vi "Gainsel.vi"(0 "Gain":enum16{"LOW", "HI", "MAX"}(ring)) -> (1 "LO":bool=TRUE, 2 "HI":bool=TRUE, 3 "MAX":bool=TRUE)   [LabVIEW 2018]
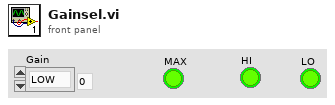
[diagram p1: front panel]
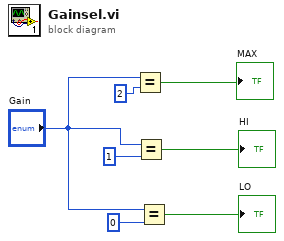
[diagram p0: block diagram]
diagram:
  n1 = Equal?(x="Gain", y=2) -> (x = y?=→"MAX":bool)
  n2 = Equal?(x="Gain", y=1) -> (x = y?=→"HI":bool)
  n3 = Equal?(x="Gain", y=0) -> (x = y?=→"LO":bool)
